vi "Instantiate Dev & RT.vi"(0 "LV Doc in":refnum<class "LV Doc.lvclass">, 5 "PID":string, 11 "error in (no error)":errorcluster) -> (4 "LV Doc in":refnum<class "LV Doc.lvclass">, 15 "error out":errorcluster)   [LabVIEW 2016, in "LV Doc.lvclass"]
uses:
  LV Doc.lvclass
  Child Classes/LV DEV/LV DEV.lvclass
  Child Classes/LV RT/LV RT.lvclass
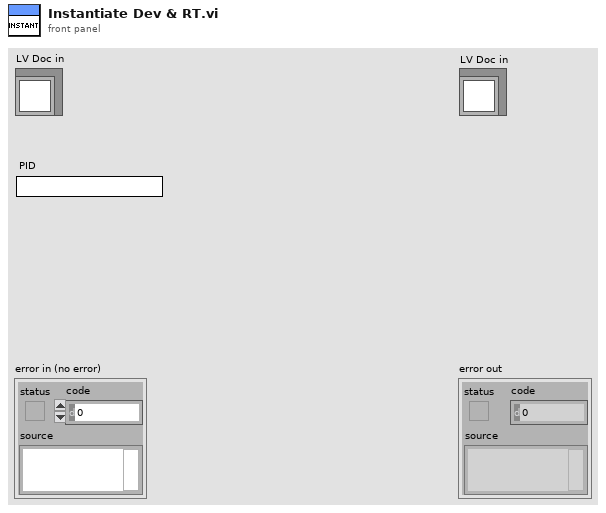
[diagram p1: front panel]
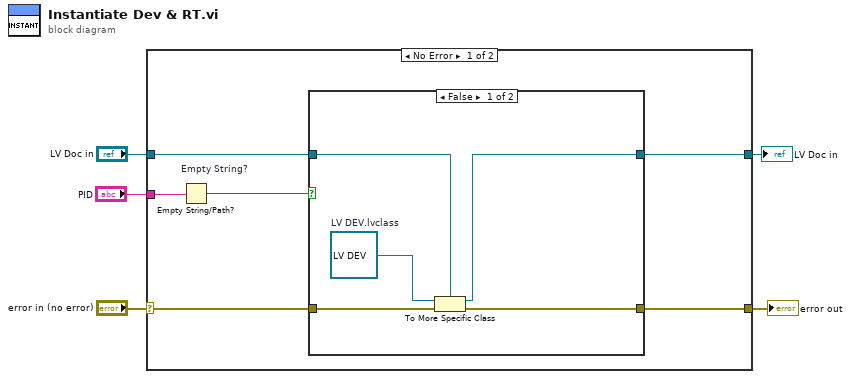
[diagram p0: block diagram]
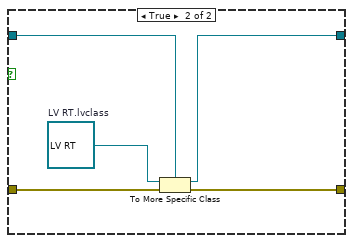
[diagram p2: hidden frame]
diagram:
  n1 = case shown="No Error" "error in (no error)" {
    selector: "error in (no error)" -> [w9 w23]
    tunnel: [w8 w23] -> w4
    tunnel: [w7 w22] -> w1
    tunnel: "LV Doc in" -> [w10 w22]
    tunnel: "PID" -> [w11 _]
    frame No Error {
      n2 = Empty String/Path? "Empty String?"(string/path=w11) -> (empty?=w6:bool)
      n3 = case shown="False" w6 {
        tunnel: [w12 w17] -> w7
        tunnel: w10 -> [w13 w18]
        tunnel: [w14 w20] -> w8
        tunnel: w9 -> [w15 w21]
        frame False {
          w16 = refnum<class "LV DEV.lvclass"> refnum  # LV DEV.lvclass
          n4 = To More Specific Class(target class=w13, reference=w16, error in=w15) -> (specific class reference=w12:refnum<class "LV Doc.lvclass">, error out=w14:errorcluster)
        }
        frame True {
          w19 = refnum<class "LV RT.lvclass"> refnum  # LV RT.lvclass
          n5 = To More Specific Class(target class=w18, reference=w19, error in=w21) -> (specific class reference=w17:refnum<class "LV Doc.lvclass">, error out=w20:errorcluster)
        }
      }
    }
    frame Error {
    }
  }
  "error out" <- w4
  "LV Doc in" <- w1
